vi "Main.vi"(8 "error in":errorcluster, 10 "Sequence Context":refnum<k7>, 11 "TestExec":refnum<class "TestExec.lvclass">) -> (0 "error out":errorcluster, 3 "TestExec":refnum<class "TestExec.lvclass">)   [LabVIEW 2019, in "Sequence Main.lvlib" / "TestExec.lvclass"]
uses:
  TestExec.lvclass
  Test Steps.ctl
  TestExec.lvclass/TestExec.ctl
  Abstract UUT/Abstract UUT.lvclass
panel:
  out "Messages":string
  out "Test Steps":T1
  out "Elapsed Time":string="0  00:01:15" caption="ms"
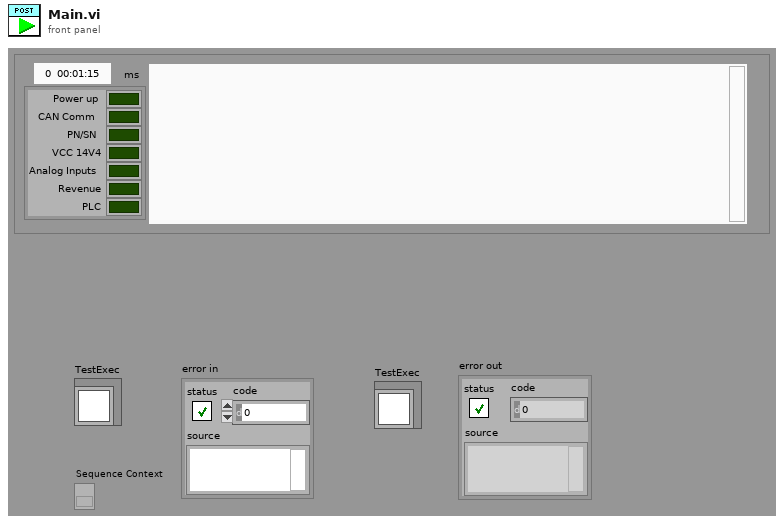
[diagram p1: front panel]
types:
  T1 = typedef "Sequence Main.lvlib/TestExec.lvclass/Test Steps.ctl" = cluster{"Power up":bool, "CAN Comm":bool, "PN/SN":bool, "VCC 14V4":bool, "Analog Inputs":bool, "Revenue":bool, "PLC":bool}
  T2 = typedef "TestStand - Status Monitor.ctl" = cluster{"Sequence Context":refnum<k7>, "Execution":refnum<k7>, "Termination Monitor":refnum<k7>}
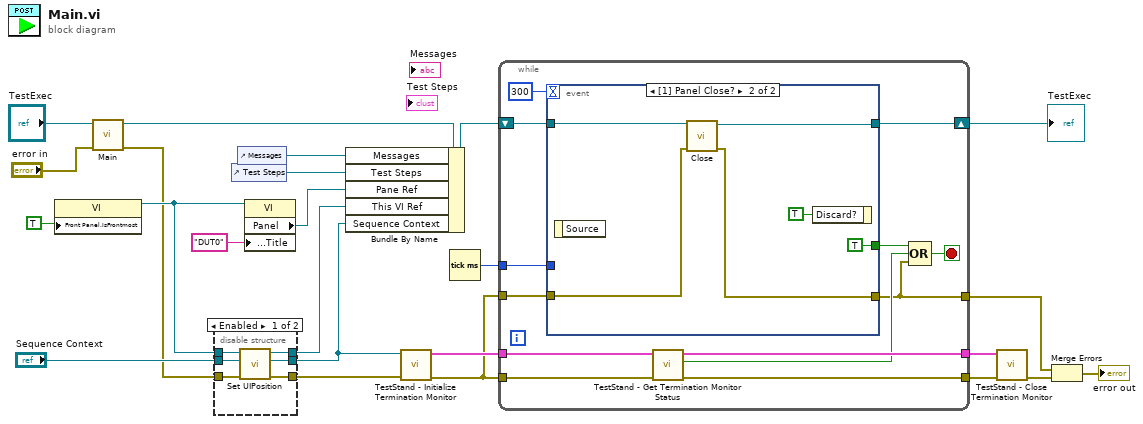
[diagram p0: block diagram]
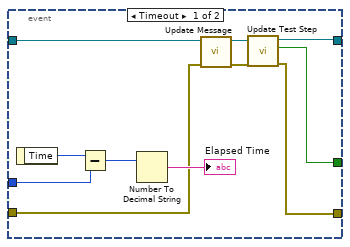
[diagram p3: hidden frame]
diagram:
  n1 = property class="VI"("Front Panel.IsFrontmost"=TRUE ("Front Panel Window:Is Frontmost")) -> (reference out=w15:refnum<vi>)  [unwired: 2 in, 1 out]
  n2 = call-parent "Main.vi"("error in"="error in", "OPC UA In"="TestExec") -> ("error out"=w8:errorcluster, "OPC UA Out"=w9:refnum<class "TestExec.lvclass">)  [unwired: 8 in]
  n3 = disable-structure shown="Enabled" {
    disable-tunnel: [w30 w31] -> w17
    disable-tunnel: "Sequence Context" -> [w26 w32]
    disable-tunnel: w15 -> [w29 w33]
    disable-tunnel: [w28 w33] -> w14
    disable-tunnel: [w25 w32] -> w13
    disable-tunnel: w8 -> [w27 w31]
    frame Enabled {
      n4 = call "Set UIPosition.vi"("error in"=w27, "Sequence Context In"=w26, "VI Ref"=w29) -> ("error out"=w30:errorcluster, "Sequence Context out"=w25:refnum<k7>, "VI Ref out"=w28:refnum<vi>)  [unwired: 6 in]
    }
    frame Disabled {
    }
  }
  n5 = control-ref of="Test Steps"() -> (w2:refnum<vi>)
  n6 = control-ref of="Messages"() -> (w1:refnum<vi>)
  n7 = property class="VI"(reference=w15, "Front Panel.Title"="DUT0" ("Front Panel Window:Title")) -> ("Panel"=w23:refnum<vi>)  [unwired: 1 in, 2 out]
  n8 = Bundle By Name(cluster=w9, "Messages"=w1, "Test Steps"=w2, "Pane Ref"=w23, "This VI Ref"=w14, "Sequence Context"=w13) -> (w4:refnum<class "TestExec.lvclass">)
  n9 = call <vilib>:"TestStand - Initialize Termination Monitor.vi"("error in (no error)"=w17, "Sequence Context In"=w13) -> ("error out"=w7:errorcluster, "Status Monitor Out"=w22:T2)  [unwired: 8 in]
  n10 = Tick Count (ms)() -> (millisecond timer value=w10:u32)
  n11 = while {
    tunnel: w7 -> [w44]
    tunnel: w22 -> [w43]
    tunnel: [w37] -> w21
    tunnel: [w41] -> w20
    tunnel: w7 -> [w36]
    tunnel: [w35] -> w11
    tunnel: w10 -> [w34]
    shift-right: [w40] -> w5
    shift-left: w4 -> [w46]
    stop <- w42 stop-if-true
    n12 = event shown="[1] Panel Close?" {
      selector: _ -> [_ _]
      dyn-events: _ -> [_ _]
      timeout: 300 -> [_ _]
      tunnel: w46 -> [w53 w63]
      tunnel: [w48 w60] -> w40
      tunnel: [w49 TRUE ("Done?")] -> w38
      tunnel: w36 -> [w47 w59]
      tunnel: [w50 w58] -> w35
      tunnel: w34 -> [w56 _]
      event Timeout {
        n13 = event-data() -> ("Time"=w57:u32)  [unwired: 1 in]
        n14 = Subtract(x=w57, y=w56) -> (x-y=w54:u32)
        n15 = Number To Decimal String(number=w54) -> (decimal integer string=→"Elapsed Time":string)  [unwired: 1 in]
        n16 = call "Update Message.vi"("error in (no error)"=w47, "TestExec in"=w53) -> ("error out"=w51:errorcluster, "TestExec out"=w52:refnum<class "TestExec.lvclass">)  [unwired: 8 in]
        n17 = call "Update Test Step.vi"("error in (no error)"=w51, "TestExec in"=w52) -> ("error out"=w50:errorcluster, "Done?"=w49:bool, "TestExec out"=w48:refnum<class "TestExec.lvclass">)  [unwired: 7 in]
      }
      event Panel Close? {
        n18 = event-data() -> ()  [unwired: 1 in, 1 out]
        n19 = call-dynamic "Close.vi"("error in (no error)"=w59, "TestExec in"=w63) -> ("error out"=w58:errorcluster, "TestExec out"=w60:refnum<class "TestExec.lvclass">)  [unwired: 8 in]
        n20 = event-data("Discard?"=TRUE) -> ()  [unwired: 1 in, 1 out]
      }
    }
    n21 = call <vilib>:"TestStand - Get Termination Monitor Status.vi"("error in (no error)"=w44, "Status Monitor In"=w43) -> ("error out"=w37:errorcluster, "Terminating or Aborting"=w39:bool, "Status Monitor Out"=w41:T2)  [unwired: 7 in]
    n22 = Compound Arithmetic op=OR(w38, w39, w35) -> (w42:bool)
  }
  "TestExec" <- w5
  n23 = call <vilib>:"TestStand - Close Termination Monitor.vi"("error in (no error)"=w21, "Status Monitor In"=w20) -> ("error out"=w18:errorcluster)  [unwired: 9 in]
  n24 = Merge Errors(w11, w18) -> (→"error out":errorcluster)
